vi "Vision Processing Cheeto.vi"(4 "error in (no error)":errorcluster, 7 "Image Size":T2=enum."320x240") -> ()   [LabVIEW 2016]
doc: "This VI runs in parallel to other tasks. It gets images from the camera, processes them for color or shape and use that information to affect robot behavior."
uses:
  <vilib>/Rock Robotics/WPI/Camera/WPI_CameraImageSize.ctl
  <vilib>/Rock Robotics/WPI/Camera/WPI_CameraWhite Balance Values.ctl
  <vilib>/Rock Robotics/WPI/Camera/WPI_CameraExposure Values.ctl
  <vilib>/Rock Robotics/WPI/Camera/WPI_CameraFrameRate.ctl
panel:
  out "x-y":u32
  in  "Boolean":bool
  out "Original Image":T1(plugin-control)
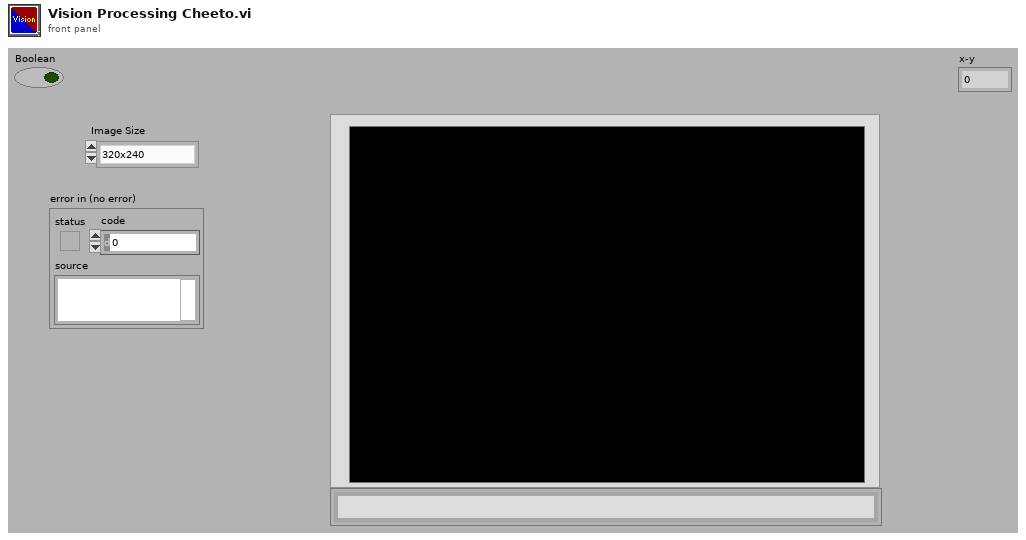
[diagram p1: front panel]
types:
  T1 = typedef "IMAQ Image.ctl" = refnum<image>
  T2 = typedef "WPI_CameraImageSize.ctl" = enum16{"640x480", "320x240", "160x120", "Custom"}
  T3 = typedef "Image Type" = u32
  T4 = typedef "WPI_CameraFrameRate.ctl" = u32
  T5 = typedef "WPI_CameraExposure Values.ctl" = enum16{"Auto", "Flicker-free 50 Hz", "Flicker-free 60 Hz", "Hold current", "Custom"}
  T6 = typedef "WPI_CameraWhite Balance Values.ctl" = enum16{"Auto", "Fixed indoor", "Fixed outdoor 1", "Fixed outdoor 2", "Fixed fluorescent 1", "Fixed fluorescent 2", "Hold current", "Custom"}
  T7 = typedef "WPI_CameraDevRef.ctl" = cluster{"Camera Address":string, "CameraStatus":errorcluster}
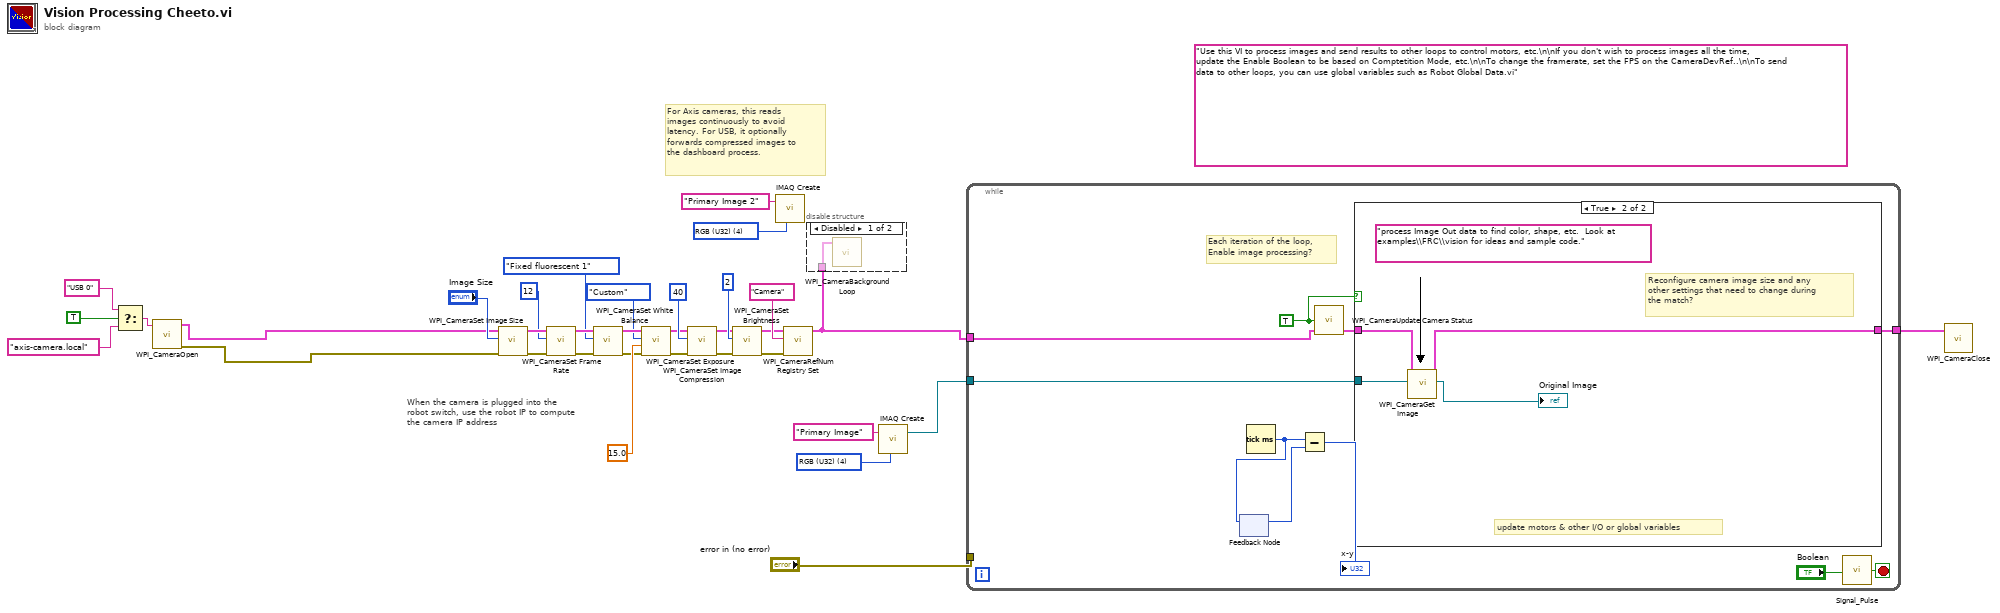
[diagram p0: block diagram]
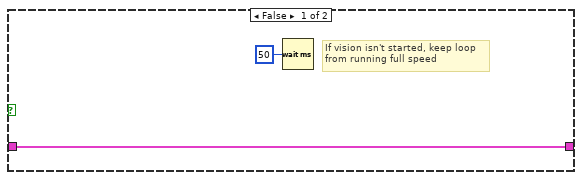
[diagram p3: hidden frame]
diagram:
  w2 = T3 4 items=["Grayscale (U8)", "Grayscale (I16)", "Grayscale (SGL)", "Complex (CSG)", "RGB (U32)", "HSL (U32)", "RGB (U64)"] ("Image Type")
  (unwired) "Use this VI to process images and send results to other loops to control motors, etc.\n\nIf you don't wish to process images all the time, update the Enable Boolean to be based on Comptetition Mode, etc.\n\nTo change the framerate, set the FPS on the CameraDevRef..\n\nTo send data to other loops, you can use global variables such as Robot Global Data.vi"
  w30 = T3 4 items=["Grayscale (U8)", "Grayscale (I16)", "Grayscale (SGL)", "Complex (CSG)", "RGB (U32)", "HSL (U32)", "RGB (U64)"] ("Image Type")
  # "When the camera is plugged into the\nrobot switch, use the robot IP to compute\nthe camera IP address"
  # "For Axis cameras, this reads\nimages continuously to avoid\nlatency. For USB, it optionally\nforwards compressed images to\nthe dashboard process."
  n1 = Select(t="USB 0" ("format string"), s=TRUE ("dot notation? (F)"), f="axis-camera.local" ("format string")) -> (s? t:f=w33:string)
  n2 = call <vilib>:"WPI_CameraOpen.vi"("Camera Address"=w33) -> ("error out"=w4:errorcluster, "CameraDevRef"=w5:T7)  [unwired: 1 in, 8 out]
  n3 = call <vilib>:"WPI_CameraSet Image Size.vi"("error in (no error)"=w4, "Image Size"="Image Size", "CameraDevRef"=w5) -> ("error out"=w18:errorcluster, "CameraDevRef Out"=w19:T7)  [unwired: 1 in, 6 out]
  n4 = call <vilib>:"WPI_CameraSet Frame Rate.vi"("error in (no error)"=w18, "Frame Rate (fps)"=T4 12, "CameraDevRef"=w19) -> ("error out"=w17:errorcluster, "CameraDevRef Out"=w21:T7)  [unwired: 7 out]
  n5 = call <vilib>:"WPI_CameraSet White Balance.vi"("error in (no error)"=w17, "White Balance"=WPI_CameraWhite_Balance_Values."Fixed fluorescent 1", "CameraDevRef"=w21) -> ("error out"=w16:errorcluster, "CameraDevRef Out"=w20:T7)  [unwired: 1 in, 6 out]
  n6 = call <vilib>:"WPI_CameraSet Exposure.vi"("error in (no error)"=w16, "Exposure (%)"=15.0, "Exposure"=WPI_CameraExposure_Values."Custom", "CameraDevRef"=w20) -> ("error out"=w15:errorcluster, "CameraDevRef Out"=w23:T7)  [unwired: 6 out]
  n7 = call <vilib>:"WPI_CameraSet Image Compression.vi"("error in (no error)"=w15, "Compression"=40, "CameraDevRef"=w23) -> ("error out"=w14:errorcluster, "CameraDevRef Out"=w22:T7)  [unwired: 7 out]
  n8 = call <vilib>:"WPI_CameraSet Brightness.vi"("error in (no error)"=w14, "Brightness"=2, "CameraDevRef"=w22) -> ("error out"=w12:errorcluster, "CameraDevRef Out"=w13:T7)  [unwired: 7 out]
  n9 = call "IMAQ Create"("Image Name"="Primary Image 2", "Image Type"=w2) -> ()  [unwired: 2 in, 3 out]
  n10 = call <vilib>:"WPI_CameraRefNum Registry Set.vi"("error in (no error)"=w12, "refnum name"="Camera", "CameraDevRef"=w13) -> ("CameraDevRef"=w1:T7)  [unwired: 1 in, 7 out]
  n11 = disable-structure shown="Disabled" {
    disable-tunnel: w1 -> [w35 _]
    frame Disabled {
      n12 = call <vilib>:"WPI_CameraBackground Loop.vi"("CameraDevRef"=w35) -> ()  [unwired: 11 in]
    }
    frame Enabled {
    }
  }
  n13 = call "IMAQ Create"("Image Name"="Primary Image", "Image Type"=w30) -> ("New Image"=w6:T1)  [unwired: 2 in, 2 out]
  n14 = while {
    tunnel: w6 -> [w44]
    tunnel: "error in (no error)" -> [_]
    tunnel: [w38] -> w7
    tunnel: w1 -> [w37]
    stop <- w36 stop-if-true
    w42 = TRUE ("Enable Vision")
    # "Each iteration of the loop,\nEnable image processing?"
    n15 = feedback #1() -> (w40:u32)  [unwired: 1 in]
    n16 = Tick Count (ms)() -> (millisecond timer value=w41:u32)
    n17 = feedback-in #1(w41) -> ()
    n18 = Subtract(x=w41, y=w40) -> (x-y=→"x-y":u32)
    n19 = call <vilib>:"WPI_CameraUpdate Camera Status.vi"("CameraDevRef In"=w37, "Enable Vision"=w42) -> ("CameraDevRef Out"=w43:T7)  [unwired: 3 in]
    n20 = case shown="True" w42 {
      tunnel: w44 -> [_ w51]
      tunnel: [w47 w48] -> w38
      tunnel: w43 -> [w47 w50]
      frame False {
        # "If vision isn't started, keep loop\nfrom running full speed"
        n21 = Wait (ms)(milliseconds to wait=u32 50) -> ()  [unwired: 1 out]
      }
      frame True {
        (unwired) "process Image Out data to find color, shape, etc.  Look at examples\\FRC\\vision for ideas and sample code."
        # "update motors & other I/O or global variables"
        # "Reconfigure camera image size and any\nother settings that need to change during\nthe match?"
        n22 = call <vilib>:"WPI_CameraGet Image.vi"("Image"=w51, "CameraDevRef"=w50) -> ("Image Out"=→"Original Image":T1, "CameraDevRef Out"=w48:T7)  [unwired: 1 in, 7 out]
      }
    }
    n23 = call <userlib>:"Signal_Pulse.vi"("Input"="Boolean") -> ("Output"=w36:bool)
  }
  n24 = call <vilib>:"WPI_CameraClose.vi"("CameraDevRef"=w7) -> ()  [unwired: 10 in, 1 out]
